vi "Create Execution Unit.vi"(8 "error in":errorcluster, 10 "Item Ref":T2=18446744073709551615 format="%.0x", 11 "Execution Unit Factory Implementation in":refnum<class "Execution Unit Factory.lvclass">) -> (0 "error out":errorcluster, 1 "Asynchronous Execution Units":T1[](array[typedef]) {"Outgoing Channels" format="%.0x"; "Incoming Channels" format="%.0x"}, 2 "Inline Execution Units":T1[](array[typedef]) {"Outgoing Channels" format="%.0x"; "Incoming Channels" format="%.0x"}, 3 "Execution Unit Factory Implementation out":refnum<class "Execution Unit Factory.lvclass">)   [LabVIEW 2020, in "Communication Bus Template Engine.lvlib" / "Implementation.lvlib" / "Execution Unit Factory.lvclass"]
uses:
  Execution Unit Factory.lvclass
  <vilib>/NI VeriStand/Custom Device API/Custom Device Item Ref.ctl
  <vilib>/NI VeriStand/Custom Device API/Custom Device API.lvlib
  NI-XNET CAN Writer Execution Unit/NI-XNET CAN Writer Execution Unit.lvclass
  Interfaces/Execution Unit/Execution Unit.lvclass
  Interfaces/Controls/Execution Unit Information.ctl
  Interfaces/Interfaces.lvlib
  NI-XNET CAN Writer Execution Unit/Parameters.ctl
  Scripting/Constants.vi
  Scripting/Communication Bus Template Scripting.lvlib
  <vilib>/NI VeriStand/Custom Device Tools/Custom Device Utility Library/Custom Device Utility Library.lvlib
  System Explorer/Implementation/System Explorer/Types/Execution Mode.ctl
  System Explorer/Implementation/Implementation.lvlib
  <vilib>/NI VeriStand/Custom Device Tools/Custom Device Utility Library/NI VeriStand - Search for All Items by GUID.vi
  <vilib>/NI VeriStand/Custom Device Tools/Custom Device Utility Library/NI VeriStand - Search for Item by GUID.vi
  C:/Dev/GitHub/niveristand-communications-bus-template/Source/Custom Device Support/Engine/Interfaces/Execution Unit/Execution Unit.lvclass
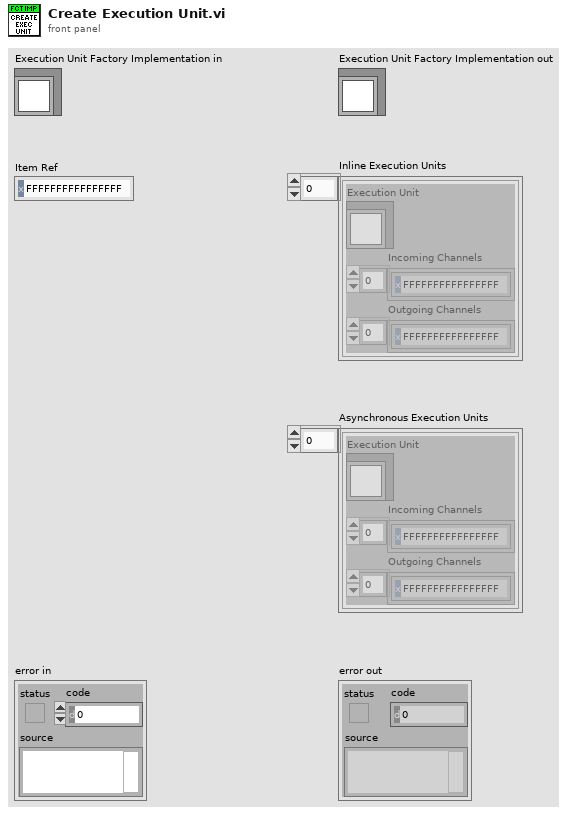
[diagram p1: front panel]
types:
  T1 = typedef "Communication Bus Template Engine.lvlib/Interfaces.lvlib/Execution Unit Information.ctl" = cluster{"Execution Unit":refnum<class "Execution Unit.lvclass">, "Incoming Channels":T2[], "Outgoing Channels":T2[]}
  T2 = typedef "Custom Device API.lvlib/Custom Device Item Ref.ctl" = u64
  T3 = typedef "Communication Bus Template System Explorer.lvlib/Implementation.lvlib/Execution Mode.ctl" = enum16{"Inline", "Asynchronous"}
  T4 = typedef "Communication Bus Template Engine.lvlib/Implementation.lvlib/NI-XNET CAN Writer Execution Unit.lvclass/Parameters.ctl" = cluster{"interface":refnum<k21>, "signal list":refnum<k21>[], "baud rate":u64}
  T5 = typedef "Communication Bus Template System Explorer.lvlib/Implementation.lvlib/XNET Interface Name.ctl" = enum16{"CAN 1", "CAN 2", "CAN 3", "CAN 4", "CAN 5", "CAN 6", "CAN 7", "CAN 8", "CAN 9", "CAN 10", "CAN 11", "CAN 12", "CAN 13", "CAN 14", "CAN 15", "CAN 16"}
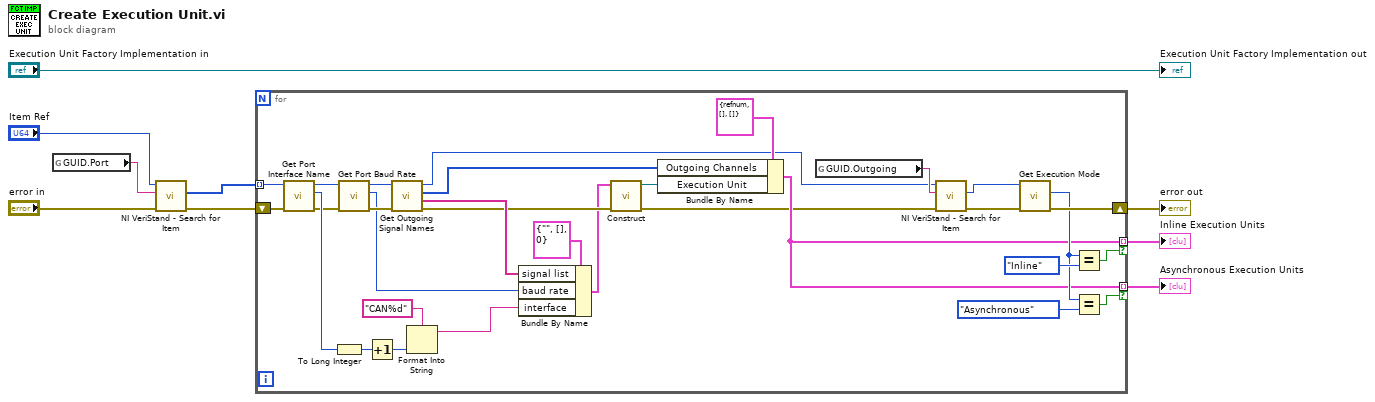
[diagram p0: block diagram]
diagram:
  n1 = global read "Constants.vi" "GUID.Port"() -> (w8:string)
  n2 = call-poly <vilib>:"NI VeriStand - Search for Item.vi"("error in"="error in", "Item GUID"=w8, "Section Ref in"="Item Ref") -> ("error out"=w6:errorcluster, "Item Refs"=w7:T2[])  [unwired: 5 in, 2 out]
  n3 = for {
    tunnel: w7 -> [w37] mode=indexing
    shift-right: [w20] -> w5
    shift-left: w6 -> [w38]
    tunnel: [w16] -> w2 mode=indexing if=w17
    tunnel: [w16] -> w1 mode=indexing if=w15
    n4 = call "Get Port Interface Name.vi"("error in"=w38, "Port Ref"=w37) -> ("error out"=w25:errorcluster, "XNET Interface Name"=w36:T5, "Port Ref out"=w26:T2)  [unwired: 7 in]
    n5 = To Long Integer(number=w36) -> (32bit integer=w35:i32)
    n6 = call "Get Port Baud Rate.vi"("error in"=w25, "Port Ref"=w26) -> ("error out"=w24:errorcluster, "Baud Rate"=w22:u32, "Port Ref out"=w23:T2)  [unwired: 7 in]
    n7 = Increment(x=w35) -> (x+1=w34:i32)
    n8 = call "Get Outgoing Signal Names.vi"("error in (no error)"=w24, "Port in"=w23) -> ("error out"=w31:errorcluster, "signal names"=w39:string[], "signals"=w28:T2[], "Port out"=w11:T2)  [unwired: 6 in]
    n9 = Format Into String(format string="CAN%d", w34) -> (resulting string=w32:string)  [unwired: 2 in, 1 out]
    n10 = Bundle By Name(cluster=T4 {"interface"="", "signal list"=[], "baud rate"=0} ("parameters"), "signal list"=w39, "baud rate"=w22, "interface"=w32) -> (w30:T4)
    n11 = call "Construct.vi"("error in (no error)"=w31, "parameters"=w30) -> ("error out"=w13:errorcluster, "NI-XNET CAN Writer Execution Unit"=w27:refnum<class "NI-XNET CAN Writer Execution Unit.lvclass">)  [unwired: 8 in]
    n12 = Bundle By Name(cluster=T1 {"Execution Unit"=refnum, "Incoming Channels"=[], "Outgoing Channels"=[]} ("Execution Unit Information"), "Outgoing Channels"=w28, "Execution Unit"=w27) -> (w16:T1)
    n13 = global read "Constants.vi" "GUID.Outgoing"() -> (w14:string)
    n14 = call-poly <vilib>:"NI VeriStand - Search for Item.vi"("error in"=w13, "Item GUID"=w14, "Section Ref in"=w11) -> ("error out"=w12:errorcluster, "Item Ref"=w10:T2)  [unwired: 5 in, 2 out]
    n15 = call "Get Execution Mode.vi"("error in"=w12, "Port Ref"=w10) -> ("error out"=w20:errorcluster, "Execution mode"=w18:T3)  [unwired: 7 in, 1 out]
    n16 = Equal?(x=w18, y=Execution_Mode."Inline") -> (x = y?=w17:bool)
    n17 = Equal?(x=w18, y=Execution_Mode."Asynchronous") -> (x = y?=w15:bool)
  }
  "error out" <- w5
  "Inline Execution Units" <- w2
  "Asynchronous Execution Units" <- w1
  "Execution Unit Factory Implementation out" <- "Execution Unit Factory Implementation in"
